vi "report results.vi"(8 "error in":errorcluster, 10 "result":refnum<class "result.lvclass">, 11 "results reporter in":refnum<class "results reporter.lvclass">) -> (0 "error out":errorcluster, 3 "results reporter out":refnum<class "results reporter.lvclass">)   [LabVIEW 2013, in "results reporter.lvclass"]
uses:
  results reporter.lvclass
  result/result.lvclass
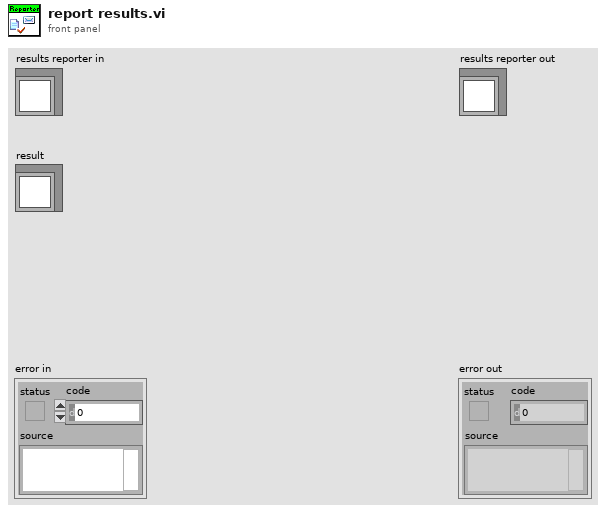
[diagram p1: front panel]
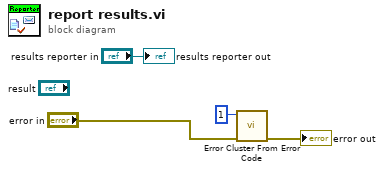
[diagram p0: block diagram]
diagram:
  n1 = call <vilib>:"Error Cluster From Error Code.vi"("error in (no error)"="error in", "error code (0)"=1) -> ("error out"=→"error out":errorcluster)  [unwired: 7 in]
  "results reporter out" <- "results reporter in"
